vi "test_ThreeSessThreePinTwoInstrTwoSiteReservation_CallGetConnectionsFromPinsForAllDcPowerPinsAllSites_ReturnsThreeConnections.vi"(8 "error in":errorcluster) -> (0 "error out":errorcluster, 2 "result":string, 3 "pass":bool)   [LabVIEW 2020, in "MeasurementServerTests.lvlib"]
uses:
  MeasurementServerTests.lvlib
  Runtime/Measurements/Measurement Plugin Session Management V1/Session Reservation/Connection.ctl
  Runtime/Measurements/Measurement Plugin Session Management V1/Session Reservation/Session Reservation.lvclass
  Runtime/Measurements/Measurement Plugin Session Management V1/Session Reservation/Connection with Session.ctl
  c3cb69a0-23cd-49fc-99d1-8c54773f0200.vi
  777eb16d-c0be-4c50-a7a6-d4611c66469e.vi
  0f44dfc3-a6fe-4b08-8e0e-634dc6c4a639.vi
  083e39de-288c-4f19-b174-41f113f7e39a.vi
  Runtime/Sessions/niDCPower Sessions/Session Factory/Session Factory.lvclass
  Runtime/Measurements/Measurement Plugin Session Management V1/Session Reservation/Pin Type.ctl
  282361f9-c062-413b-9df1-ec4b2bd2456d.vi
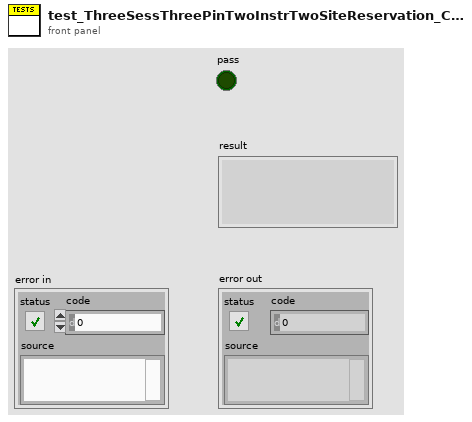
[diagram p1: front panel]
types:
  T1 = typedef "Measurement Plugin Session Management V1.lvlib/Session Reservation.lvclass/Pin Type.ctl" = enum16{"DUT and System Pins", "System Pins"}
  T2 = typedef "Measurement Plugin Session Management V1.lvlib/Session Reservation.lvclass/Connection.ctl" = cluster{"pin or relay name":string, "site":i32, "instrument type id":string, "channel":string}
  T3 = typedef "Measurement Plugin Session Management V1.lvlib/Session Reservation.lvclass/Connection with Session.ctl" = cluster{"connection":T2, "session":variant}
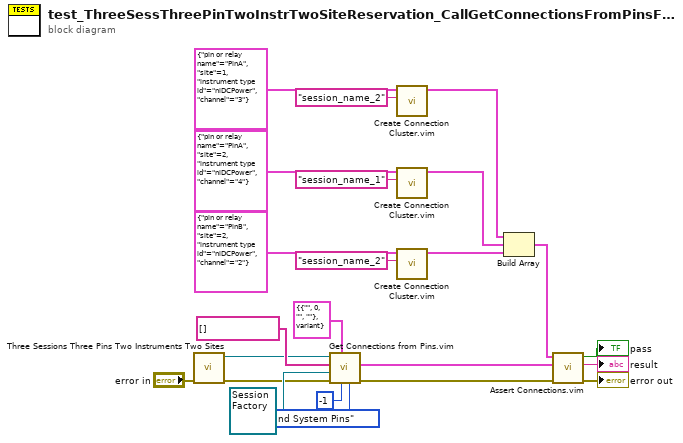
[diagram p0: block diagram]
diagram:
  n1 = call "Three Sessions Three Pins Two Instruments Two Sites.vi"("error in"="error in") -> ("error out"=w3:errorcluster, "session reservation out"=w4:refnum<class "Session Reservation.lvclass">)  [unwired: 8 in, 1 out]
  n2 = call "Get Connections from Pins.vim"("pin type"=Pin_Type."DUT and System Pins", "site"=-1, "connection type"=T3 {"connection"={"pin or relay name"="", "site"=0, "instrument type id"="", "channel"=""}, "session"=variant} ("connection"), "error in"=w3, "session factory"=refnum<class "Session Factory.lvclass"> refnum ("MeasurementLink niDCPower.lvlib:Instrument.lvclass"), "pin or relay names"=string[] [], "session reservation in"=w4) -> ("error out"=w2:errorcluster, "connections"=w21:T3[])  [unwired: 2 in, 1 out]
  n3 = call "Create Connection Cluster.vim"("session in"="session_name_2", "hardware independent connection in"=T2 {"pin or relay name"="PinA", "site"=1, "instrument type id"="niDCPower", "channel"="3"} ("connection")) -> ("connection out"=w17:T3)  [unwired: 9 in]
  n4 = call "Create Connection Cluster.vim"("session in"="session_name_1", "hardware independent connection in"=T2 {"pin or relay name"="PinA", "site"=2, "instrument type id"="niDCPower", "channel"="4"} ("connection")) -> ("connection out"=w16:T3)  [unwired: 9 in]
  n5 = call "Create Connection Cluster.vim"("session in"="session_name_2", "hardware independent connection in"=T2 {"pin or relay name"="PinB", "site"=2, "instrument type id"="niDCPower", "channel"="2"} ("connection")) -> ("connection out"=w15:T3)  [unwired: 9 in]
  n6 = Build Array(w17, w16, w15) -> (w14:T3[])
  n7 = call "Assert Connections.vim"("error in"=w2, "actual connections"=w21, "expected connections"=w14) -> ("error out"=→"error out":errorcluster, "result"=→"result":string, "pass"=→"pass":bool)  [unwired: 6 in]
